vi "UI_Elmt_Visible(Label).vi"(8 "error in (no error)":errorcluster, 9 "Visible":bool, 10 "Elmt Label":string, 11 "UI_Actor in":refnum<class "UI_Actor.lvclass">) -> (0 "error out":errorcluster, 1 "Found":bool, 3 "UI_Actor out":refnum<class "UI_Actor.lvclass">)   [LabVIEW 2020, in "UI_Actor.lvlib" / "UI_Actor.lvclass"]
doc: "Accès à un élément par son label.\n<b> NEVER USE IN FOR LOOP </b> \nLa ref est stockée au premier appel en fgv.\nLe VI doit etre dédié à un unique élement."
uses:
  UI_Actor.lvclass
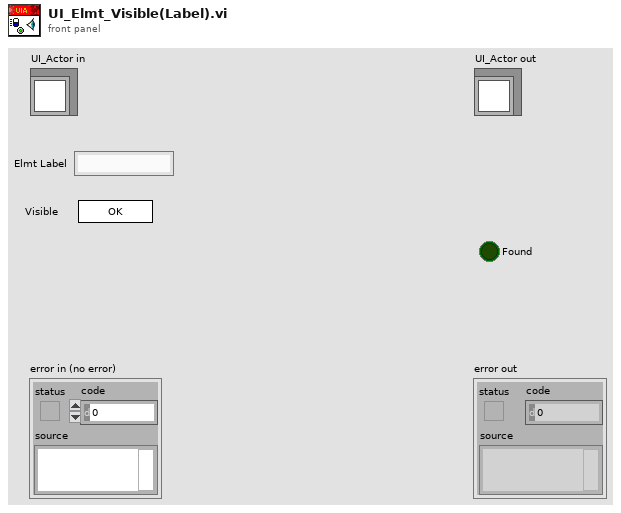
[diagram p1: front panel]
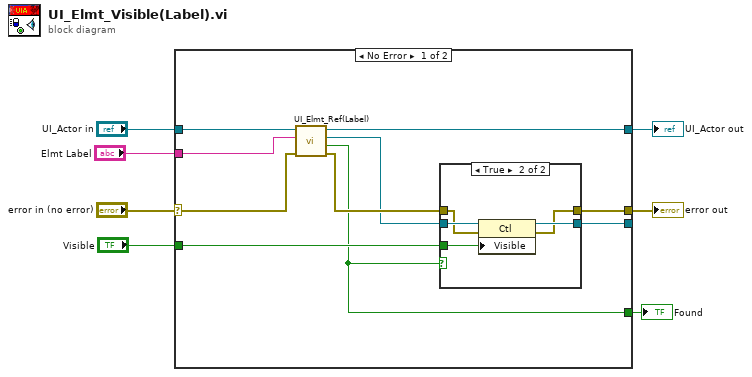
[diagram p0: block diagram]
diagram:
  n1 = case shown="No Error" "error in (no error)" {
    selector: "error in (no error)" -> [w12 w26]
    tunnel: [w14 w26] -> w6
    tunnel: [w16 w25] -> w4
    tunnel: "UI_Actor in" -> [w17 w25]
    tunnel: "Elmt Label" -> [w15 _]
    tunnel: [w13 _] -> _
    tunnel: [w8 _] -> w2
    tunnel: "Visible" -> [w11 _]
    frame No Error {
      n2 = call "UI_Elmt_Ref(Label).vi"("error in (no error)"=w12, "Elmt Label"=w15, "UI_Actor in"=w17) -> ("error out"=w10:errorcluster, "Found"=w8:bool, "Ctl Refnum"=w9:refnum<vi>, "UI_Actor out"=w16:refnum<class "UI_Actor.lvclass">)  [unwired: 5 in]
      n3 = case shown="True" w8 {
        tunnel: [w19 w24] -> w13
        tunnel: w9 -> [w19 w23]
        tunnel: w11 -> [_ w22]
        tunnel: w10 -> [w18 w21]
        tunnel: [w18 w20] -> w14
        frame False {
        }
        frame True {
          n4 = property class="Ctl"(reference=w23, error in=w21, "Visible"=w22) -> (reference out=w24:refnum<vi>, error out=w20:errorcluster)
        }
      }
    }
    frame Error {
    }
  }
  "error out" <- w6
  "UI_Actor out" <- w4
  "Found" <- w2
